vi "test.vi"() -> ()   [LabVIEW 2013]
panel:
  in  "Software Loop Rate (ms)":u32=100
  in  "Stop":bool
  in  "Duty Cycle (%)":dbl[](array[numeric])
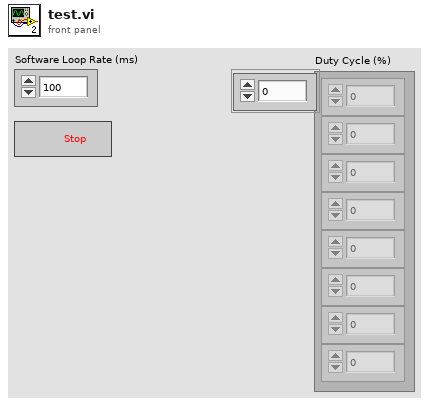
[diagram p1: front panel]
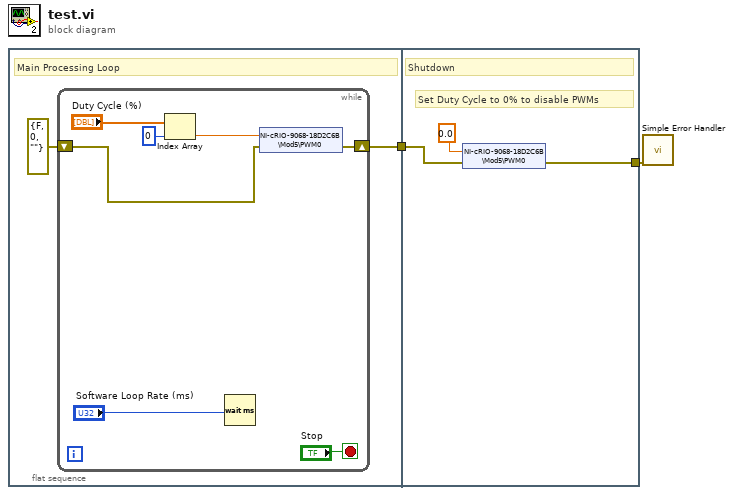
[diagram p0: block diagram]
diagram:
  n1 = flat-sequence {
    tunnel: [w4] -> w2
    tunnel: w2 -> [w12]
    tunnel: [w13] -> w1
    frame #0 {
      # "Main Processing Loop"
      n2 = while {
        shift-right: [w7] -> w4
        shift-left: errorcluster {"status"=FALSE, "code"=0, "source"=""} ("error IO") -> [w5]
        stop <- "Stop" stop-if-true
        n3 = Index Array(array="Duty Cycle (%)", index=0) -> (element=w8:dbl)
        n4 = Wait (ms)(milliseconds to wait="Software Loop Rate (ms)") -> ()  [unwired: 1 out]
        n5 = shared-variable "NI-cRIO-9068-18D2C6B\\Mod5\\PWM0"(w8, error in=w5) -> (error out=w7:errorcluster)
      }
    }
    frame #1 {
      # "Set Duty Cycle to 0% to disable PWMs"
      # "Shutdown"
      n6 = shared-variable "NI-cRIO-9068-18D2C6B\\Mod5\\PWM0"(0.0 ("1 Hz"), error in=w12) -> (error out=w13:errorcluster)
    }
  }
  n7 = call <vilib>:"Simple Error Handler.vi"("error in (no error)"=w1) -> ()  [unwired: 1 in, 8 out]
